vi "Determine Type.vi"(11 "Hand":string) -> (3 "Type":T1(ring))   [LabVIEW 2021]
uses:
  <userlib>/_OpenG.lib/array/array.llb/Remove Duplicates from 1D Array (U8)__ogtk.vi
  <userlib>/_OpenG.lib/array/array.llb/Index 1D Array Elements (U8)__ogtk.vi
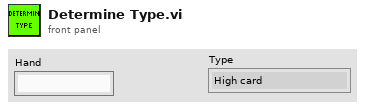
[diagram p1: front panel]
types:
  T1 = enum16{"High card", "One pair", "Two pair", "Three of a kind", "Full house", "Four of a kind", "Five of a kind"}
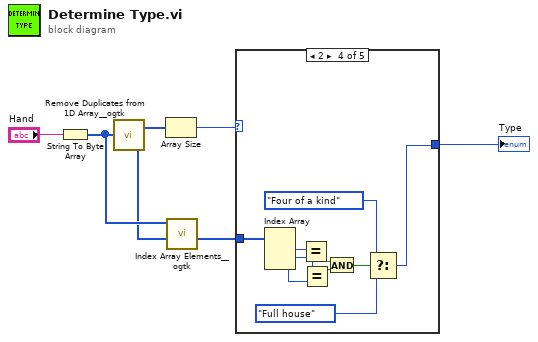
[diagram p0: block diagram]
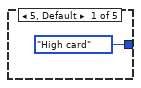
[diagram p2: hidden frame]
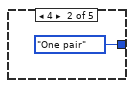
[diagram p3: hidden frame]
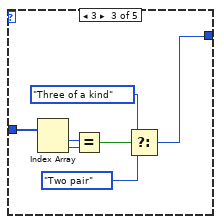
[diagram p4: hidden frame]
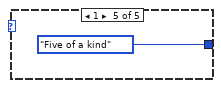
[diagram p5: hidden frame]
diagram:
  n1 = String To Byte Array(string="Hand") -> (unsigned byte array=w3:u8[])
  n2 = call-poly <userlib>:"Remove Duplicates from 1D Array__ogtk.vi"("Input Array"=w3) -> ("Output Array"=w6:u8[], "indices of removed elements"=w2:i32[])
  n3 = Array Size(array=w6) -> (size(s)=w5:i32)
  n4 = call-poly <userlib>:"Index Array Elements__ogtk.vi"("indices"=w2, "array"=w3) -> ("elements"=w1:u8[])  [unwired: 9 in]
  n5 = case shown="2" w5 {
    tunnel: [T1."High card" ("Type") T1."One pair" ("Type") w10 w24 T1."Five of a kind" ("Type")] -> w4
    tunnel: w1 -> [_ _ w16 w26 _]
    frame 5, Default {
    }
    frame 4 {
    }
    frame 3 {
      n6 = Index Array(array=w16) -> (element #1=w14:u8, element #2=w15:u8)  [unwired: 2 in]
      n7 = Equal?(x=w14, y=w15) -> (x = y?=w13:bool)
      n8 = Select(t=T1."Three of a kind" ("Type"), s=w13, f=T1."Two pair" ("Type")) -> (s? t:f=w10:T1)
    }
    frame 2 {
      n9 = Index Array(array=w26) -> (element #1=w25:u8, element #2=w22:u8, element #3=w21:u8)  [unwired: 3 in]
      n10 = Equal?(x=w25, y=w22) -> (x = y?=w19:bool)
      n11 = Equal?(x=w22, y=w21) -> (x = y?=w20:bool)
      n12 = And(x=w19, y=w20) -> (x .and. y?=w18:bool)
      n13 = Select(t=T1."Four of a kind" ("Type"), s=w18, f=T1."Full house" ("Type")) -> (s? t:f=w24:T1)
    }
    frame 1 {
    }
  }
  "Type" <- w4
